vi "Write Socket.lvclass.vi"(8 "error in (no error)":errorcluster, 10 "Socket.lvclass":refnum<class "Socket.lvclass">, 11 "Communication Manager in":refnum<class "Communication Manager.lvclass">) -> (0 "error out":errorcluster, 3 "Communication Manager out":refnum<class "Communication Manager.lvclass">)   [LabVIEW 2018, in "Communication Manager.lvclass"]
uses:
  Communication Manager.lvclass
  Socket/Socket.lvclass
  Communication Manager.lvclass/Communication Manager.ctl
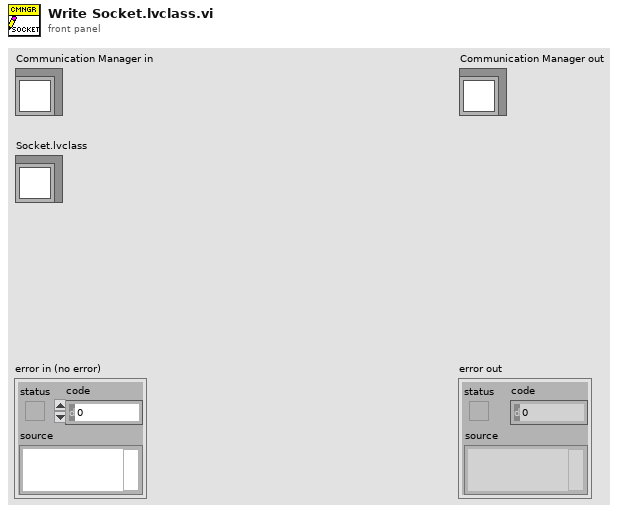
[diagram p1: front panel]
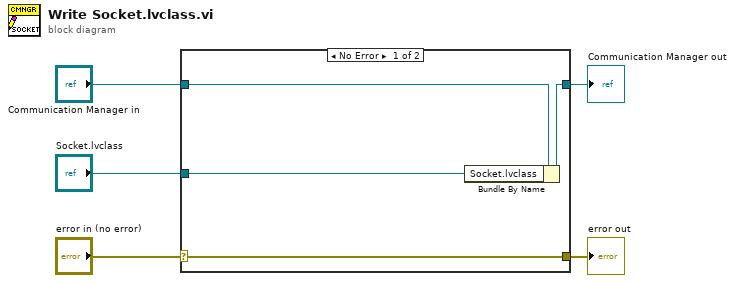
[diagram p0: block diagram]
diagram:
  n1 = case shown="No Error" "error in (no error)" {
    selector: "error in (no error)" -> [w9 w10]
    tunnel: [w9 w10] -> w4
    tunnel: [w7 w11] -> w2
    tunnel: "Communication Manager in" -> [w8 w11]
    tunnel: "Socket.lvclass" -> [w6 _]
    frame No Error {
      n2 = Bundle By Name(cluster=w8, "Socket.lvclass"=w6) -> (w7:refnum<class "Communication Manager.lvclass">)
    }
    frame Error {
    }
  }
  "error out" <- w4
  "Communication Manager out" <- w2
